vi "clm.config.build-path.vi"(9 "Proc Name":string, 10 "Section Name":string, 11 "Module Name":string) -> (3 "Relative Path":string)   [LabVIEW 2024]
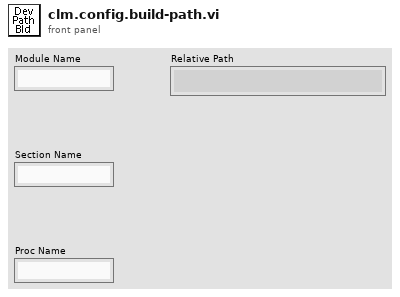
[diagram p1: front panel]
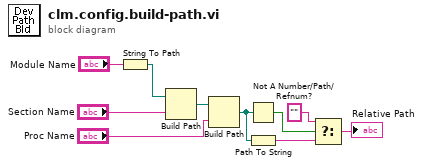
[diagram p0: block diagram]
diagram:
  n1 = String To Path(string="Module Name") -> (path=w1:path)
  n2 = Build Path(base path=w1, name or relative path="Section Name") -> (appended path=w10:path)
  n3 = Build Path(base path=w10, name or relative path="Proc Name") -> (appended path=w6:path)
  n4 = Not A Number/Path/Refnum?(number/path/refnum=w6) -> (NaN/Path/Refnum?=w5:bool)
  n5 = Path To String(path=w6) -> (string=w4:string)
  n6 = Select(t="", s=w5, f=w4) -> (s? t:f=→"Relative Path":string)
